vi "Configure Detector Mode.vi"(8 "error in (no error)":errorcluster, 10 "Detector Mode":T1(ring), 11 "MXA in":refnum<class "MXA.lvclass">) -> (0 "error out":errorcluster, 3 "MXA out":refnum<class "MXA.lvclass">)   [LabVIEW 2020, in "MXA.lvclass"]
uses:
  MXA.lvclass
  C:/Sandbox/Git_Sandbox/WiSpry Test Framework source code (LV20)/WiSpry Test Framework/Instruments/Instrument.lvclass
  Instrument.lvclass/Instrument.ctl
  Instrument.lvclass
  <instrlib>/Agilent MXA Series/Agilent MXA Series.lvlib
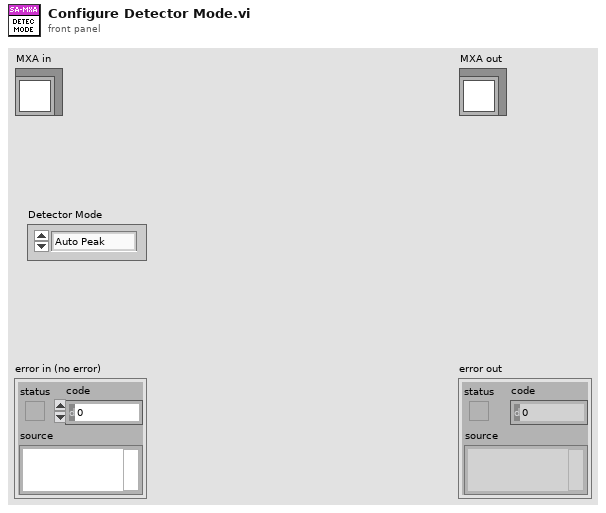
[diagram p1: front panel]
types:
  T1 = enum16{"Auto Peak", "Negative Peak", "Positive Peak", "Quasipeak", "Sample", "RMS", "Average", "CISPR Average", "CISPR RMS"}
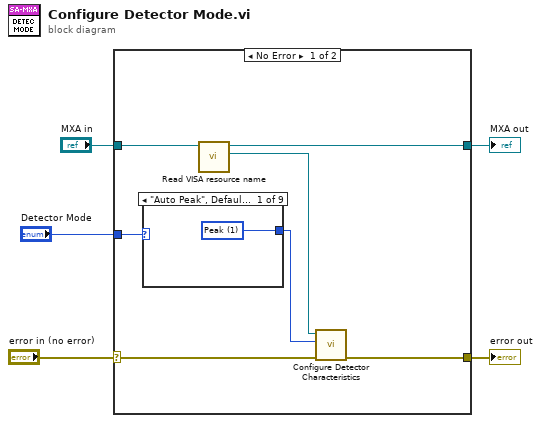
[diagram p0: block diagram]
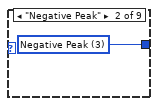
[diagram p2: hidden frame]
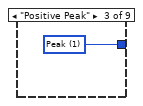
[diagram p3: hidden frame]
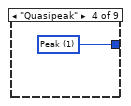
[diagram p4: hidden frame]
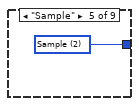
[diagram p5: hidden frame]
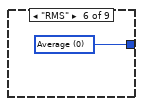
[diagram p6: hidden frame]
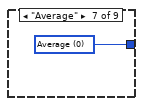
[diagram p7: hidden frame]
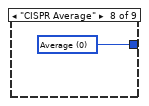
[diagram p8: hidden frame]
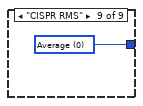
[diagram p9: hidden frame]
diagram:
  n1 = case shown="No Error" "error in (no error)" {
    selector: "error in (no error)" -> [w9 w23]
    tunnel: "MXA in" -> [w12 w22]
    tunnel: [w8 w23] -> w5
    tunnel: [w11 w22] -> w3
    tunnel: "Detector Mode" -> [w7 _]
    frame No Error {
      n2 = case shown="\"Auto Peak\", Default" w7 {
        tunnel: [w13 w14 w15 w16 w17 w18 w19 w20 w21] -> w6
        frame "Auto Peak", Default {
          w13 = 1 items=["Average", "Peak", "Sample", "Negative Peak", "Normal"] ("Manual Offset Detector Type (0: Average)")
        }
        frame "Negative Peak" {
          w14 = 3 items=["Average", "Peak", "Sample", "Negative Peak", "Normal"] ("Manual Offset Detector Type (0: Average)")
        }
        frame "Positive Peak" {
          w15 = 1 items=["Average", "Peak", "Sample", "Negative Peak", "Normal"] ("Manual Offset Detector Type (0: Average)")
        }
        frame "Quasipeak" {
          w16 = 1 items=["Average", "Peak", "Sample", "Negative Peak", "Normal"] ("Manual Offset Detector Type (0: Average)")
        }
        frame "Sample" {
          w17 = 2 items=["Average", "Peak", "Sample", "Negative Peak", "Normal"] ("Manual Offset Detector Type (0: Average)")
        }
        frame "RMS" {
          w18 = 0 items=["Average", "Peak", "Sample", "Negative Peak", "Normal"] ("Manual Offset Detector Type (0: Average)")
        }
        frame "Average" {
          w19 = 0 items=["Average", "Peak", "Sample", "Negative Peak", "Normal"] ("Manual Offset Detector Type (0: Average)")
        }
        frame "CISPR Average" {
          w20 = 0 items=["Average", "Peak", "Sample", "Negative Peak", "Normal"] ("Manual Offset Detector Type (0: Average)")
        }
        frame "CISPR RMS" {
          w21 = 0 items=["Average", "Peak", "Sample", "Negative Peak", "Normal"] ("Manual Offset Detector Type (0: Average)")
        }
      }
      n3 = call "Read VISA resource name.vi"("Instrument in"=w12) -> ("VISA resource name"=w10:refnum<visa-resource-name>, "Instrument out"=w11:refnum<class "MXA.lvclass">)  [unwired: 9 in]
      n4 = call <instrlib>:"Configure Detector Characteristics.vi"("error in (no error)"=w9, "Manual Offset Detector Type (0: Average)"=w6, "VISA resource name"=w10) -> ("error out"=w8:errorcluster)  [unwired: 7 in, 1 out]
    }
    frame Error {
    }
  }
  "error out" <- w5
  "MXA out" <- w3
